vi "Input_Sensors_TipperV2.vi"() -> (0 "error out":T1, 3 "Tipper Inputs":T2)   [LabVIEW 2011]
uses:
  Inputs_Sensors_TipperV2.ctl
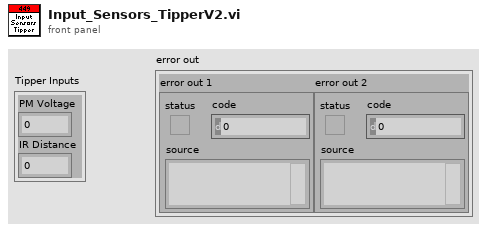
[diagram p1: front panel]
types:
  T1 = cluster{"error out 1":errorcluster, "error out 2":errorcluster}
  T2 = typedef "Inputs_Sensors_TipperV2.ctl" = cluster{"PM Voltage":dbl, "IR Distance":dbl}
  T3 = typedef "WPI_AnalogChannelDevRef.ctl" = cluster{"DevStatus":errorcluster, "Analog Module":T4, "Analog Channel":T5}
  T4 = typedef "FPGA_TypedefAnalogModule.ctl" = enum16{"Analog Module 1", "Analog Module 2"}
  T5 = typedef "FPGA_AIChannel.ctl" = enum8{"AI 1", "AI 2", "AI 3", "AI 4", "AI 5", "AI 6", "AI 7", "AI 8", "Invalid"}
  T6 = cluster{"error out":errorcluster, "error out":errorcluster}
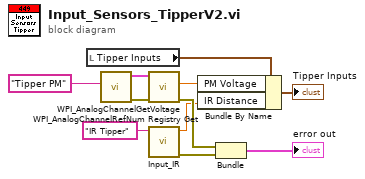
[diagram p0: block diagram]
diagram:
  n1 = local read "Tipper Inputs"() -> (w6:T2)
  n2 = call <vilib>:"WPI_AnalogChannelRefNum Registry Get.vi"("refnum name"="Tipper PM") -> ("error out"=w9:errorcluster, "AIDeviceRef"=w10:T3)  [unwired: 9 in]
  n3 = call <vilib>:"WPI_AnalogChannelGetVoltage.vi"("error in (no error)"=w9, "AIDeviceRef"=w10) -> ("error out"=w5:errorcluster, "Voltage"=w7:dbl)  [unwired: 7 in, 1 out]
  n4 = call "Input_IR.vi"("Reference Name"="IR Tipper" ("refnum name")) -> ("error out"=w2:errorcluster, "Distance (in)"=w3:dbl)  [unwired: 9 in]
  n5 = Bundle By Name(cluster=w6, "PM Voltage"=w7, "IR Distance"=w3) -> (→"Tipper Inputs":T2)
  n6 = Bundle("error out"=w5, "error out"=w2) -> (→"error out":T6)  [unwired: 1 in]
